vi "Query Marker.vi"(8 "error in (no error)":errorcluster, 10 "Marker Number":u8=1, 11 "VNA-ZNB in":refnum<class "VNA-ZNB.lvclass">) -> (0 "error out":errorcluster, 1 "Data":dbl, 2 "Frequency":dbl, 3 "VNA-ZNB out":refnum<class "VNA-ZNB.lvclass">)   [LabVIEW 2020, in "VNA-ZNB.lvclass"]
doc: "Query the marker on the active trace"
uses:
  VNA-ZNB.lvclass
  C:/Sandbox/Git_Sandbox/WiSpry Test Framework source code (LV20)/WiSpry Test Framework/Instruments/Instrument.lvclass
  Instrument.lvclass/Instrument.ctl
  Instrument.lvclass
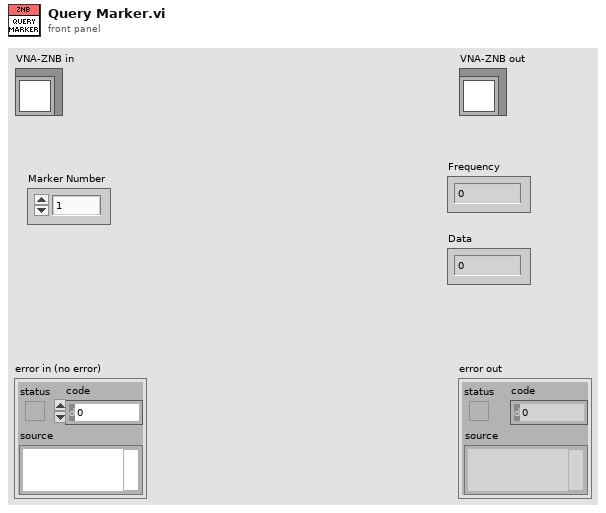
[diagram p1: front panel]
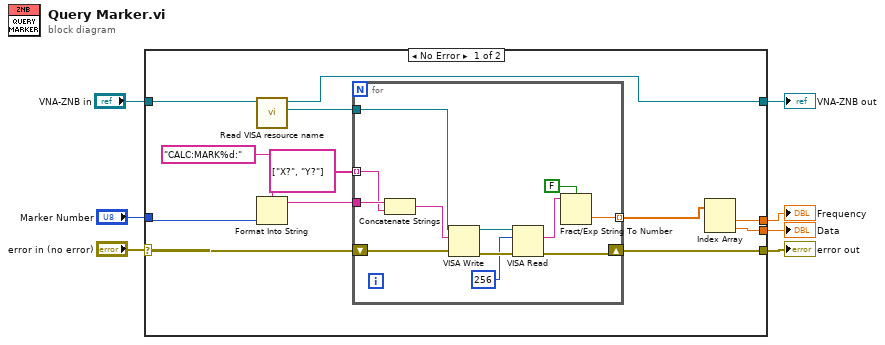
[diagram p0: block diagram]
diagram:
  n1 = case shown="No Error" "error in (no error)" {
    selector: "error in (no error)" -> [w16 w32]
    tunnel: "Marker Number" -> [w18 _]
    tunnel: "VNA-ZNB in" -> [w14 w33]
    tunnel: [w12 w33] -> w1
    tunnel: [w10 _] -> w4
    tunnel: [w9 _] -> w3
    tunnel: [w8 w32] -> w2
    frame No Error {
      n2 = call "Read VISA resource name.vi"("Instrument in"=w14) -> ("VISA resource name"=w13:refnum<visa-resource-name>, "Instrument out"=w12:refnum<class "VNA-ZNB.lvclass">)  [unwired: 9 in]
      n3 = Format Into String(format string="CALC:MARK%d:", w18) -> (resulting string=w17:string)  [unwired: 2 in, 1 out]
      n4 = for {
        tunnel: w17 -> [w31]
        shift-right: [w26] -> w8
        shift-left: w16 -> [w29]
        tunnel: string[] ["X?", "Y?"] -> [w30] mode=indexing
        tunnel: w13 -> [w28]
        tunnel: [w20] -> w11 mode=indexing
        n5 = Concatenate Strings(w31, w30) -> (w27:string)
        n6 = VISA Write(VISA resource name=w28, write buffer=w27, error in (no error)=w29) -> (VISA resource name out=w24:refnum<visa-resource-name>, error out=w25:errorcluster)  [unwired: 1 out]
        n7 = VISA Read(VISA resource name=w24, byte count=u32 256, error in (no error)=w25) -> (read buffer=w22:string, error out=w26:errorcluster)  [unwired: 2 out]
        n8 = Fract/Exp String To Number(use system decimal point (T)=FALSE, string=w22) -> (number=w20:dbl)  [unwired: 2 in, 1 out]
      }
      n9 = Index Array(array=w11) -> (element #1=w10:dbl, element #2=w9:dbl)  [unwired: 2 in]
    }
    frame Error {
    }
  }
  "error out" <- w2
  "VNA-ZNB out" <- w1
  "Data" <- w3
  "Frequency" <- w4
